vi "sub vi - AI USB4704 (3) v73.vi"(0 "Task0":i32, 1 "Test":bool, 5 "Task1":i32, 7 "Task2":i32, 11 "SAMPLES":dbl, 12 "Max Errors":i32=10, 13 "MAIL SETTINGS":T1) -> (3 "Fault":bool, 4 "data 0":waveform(dbl)[](array[waveform]), 6 "data 1":waveform(dbl)[](array[waveform]), 8 "data 2":waveform(dbl)[](array[waveform]), 10 "loop time":dbl format="%.6g", 14 "Fault Counts":i32[](array[numeric]), 15 "error array":errorcluster[](array[cluster]))   [LabVIEW 2017]
uses:
  <userlib>/DAQNavi Polymorphic VI/read/DAQNavi Read (Analog 1D Wfm NChan NSamp).vi
panel:
  in  "File Path":path
  out "Fault 3":bool
  out "Fault 2":bool
  out "Fault 1":bool
  out "String":string
  in  "Tab Control":enum32{"USB #0", "USB #1", "USB #2"}(tab)
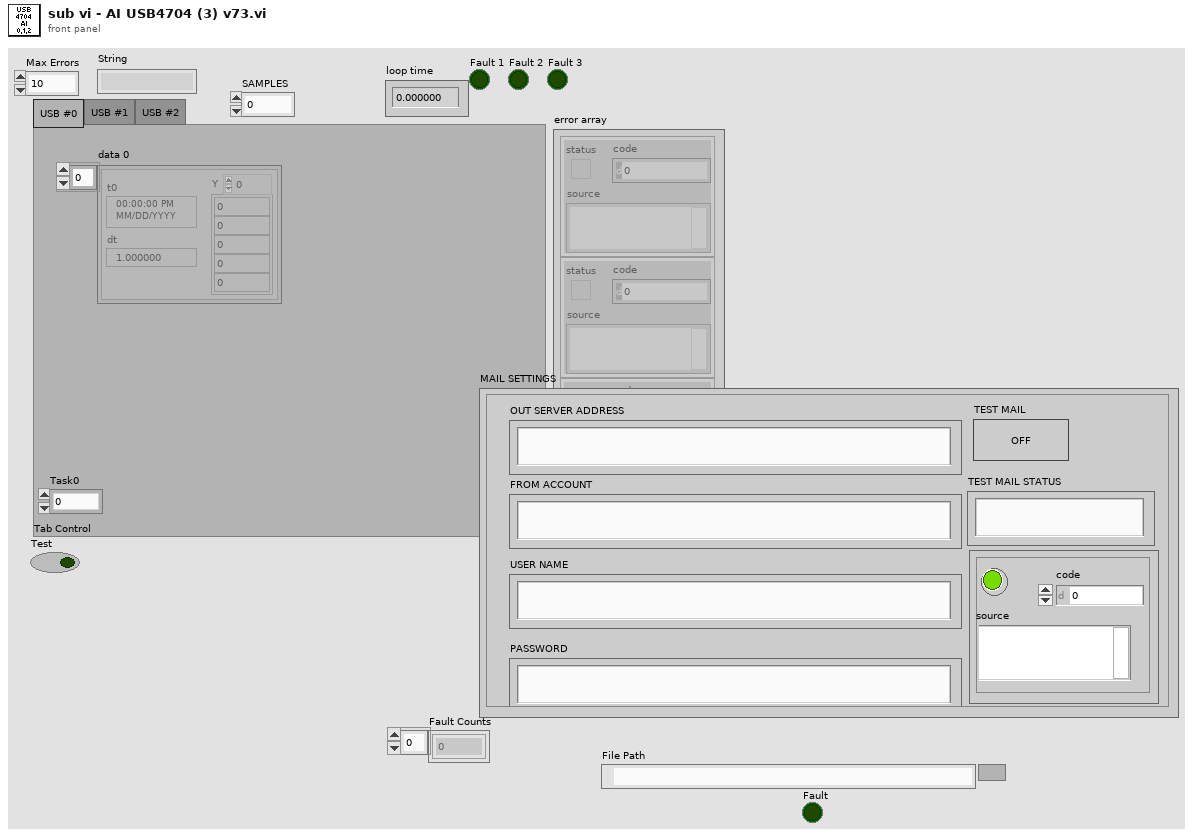
[diagram p1: front panel]
types:
  T1 = cluster{"OUT SERVER ADDRESS":string, "FROM ACCOUNT":string, "USER NAME":string, "PASSWORD":string, "TEST MAIL":bool, "TEST MAIL STATUS":string, "mail error":errorcluster}
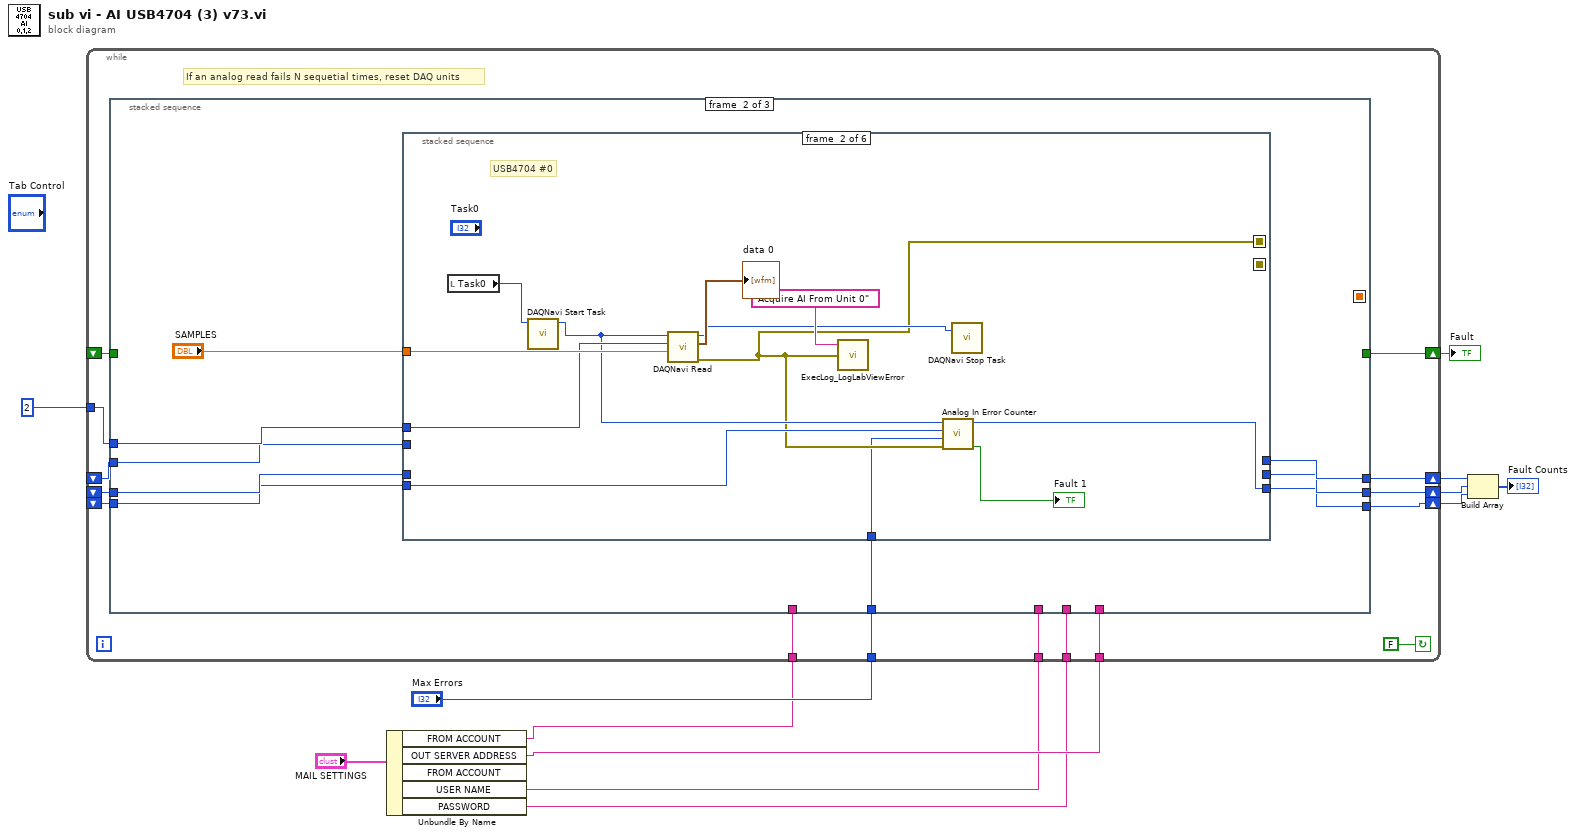
[diagram p0: block diagram]
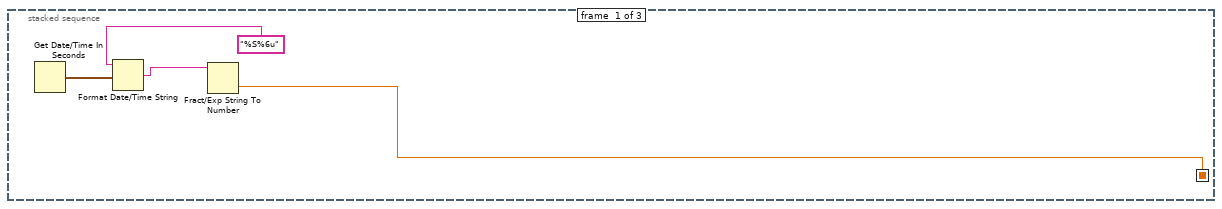
[diagram p2: hidden frame]
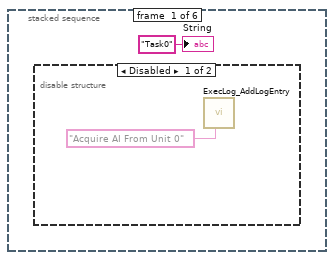
[diagram p3: hidden frame]
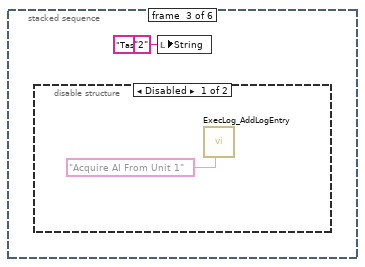
[diagram p5: hidden frame]
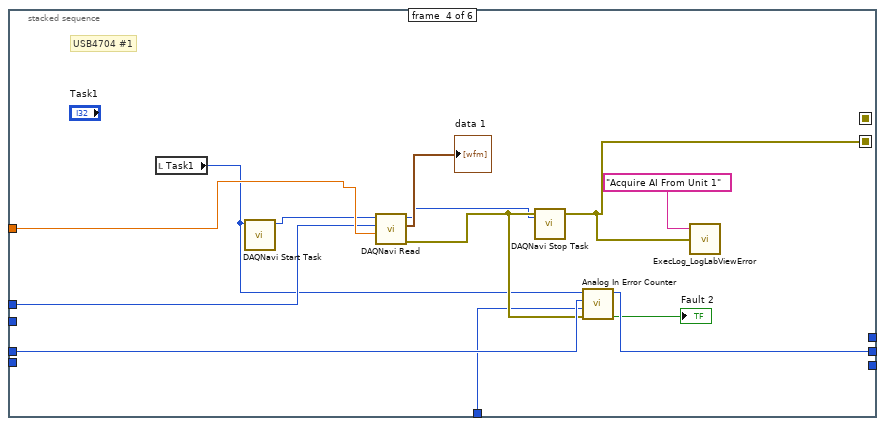
[diagram p7: hidden frame]
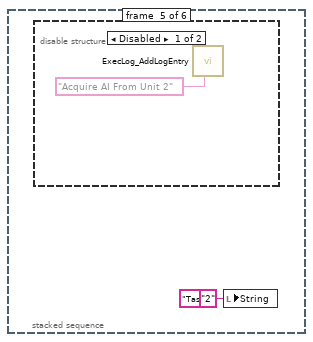
[diagram p8: hidden frame]
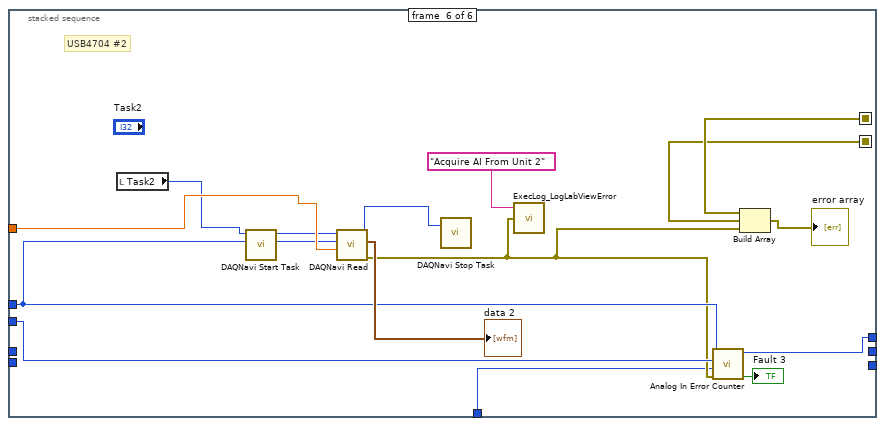
[diagram p10: hidden frame]
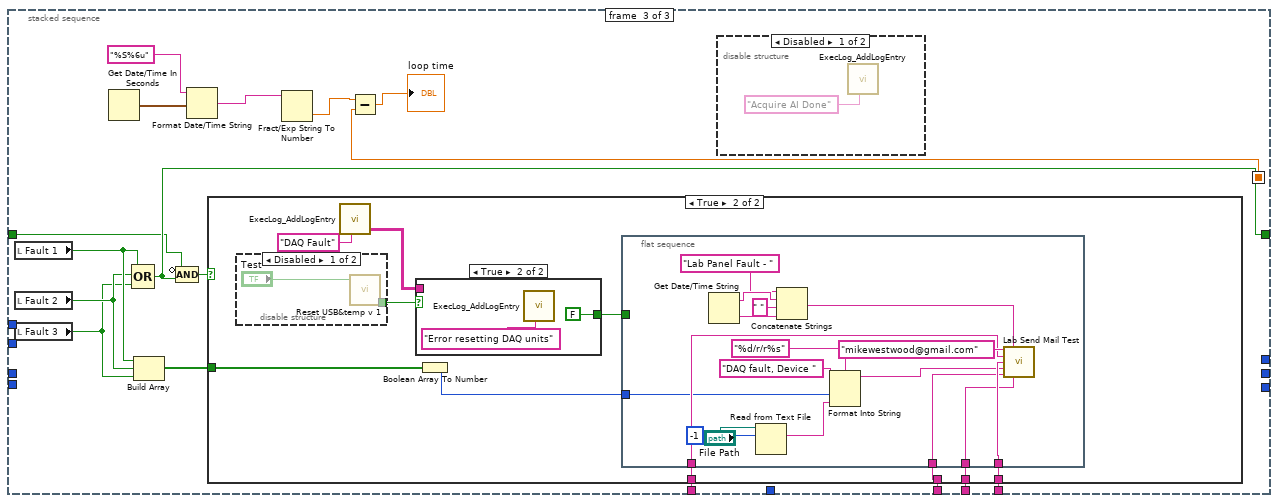
[diagram p11: hidden frame]
diagram:
  n1 = Unbundle By Name("MAIL SETTINGS") -> ("FROM ACCOUNT"=w8:string, "OUT SERVER ADDRESS"=w9:string, "USER NAME"=w7:string, "PASSWORD"=w6:string)  [unwired: 1 out]
  n2 = while {
    tunnel: 2 -> [w27]
    shift-right: [w26] -> w5
    shift-left: _ -> [w25]
    shift-right: [w23] -> w4
    shift-left: _ -> [w24]
    shift-right: [w21] -> w3
    shift-left: _ -> [w22]
    tunnel: "Max Errors" -> [w19]
    tunnel: w9 -> [w18]
    tunnel: w8 -> [w17]
    tunnel: w7 -> [w16]
    tunnel: w6 -> [w15]
    shift-right: [w14] -> w1
    shift-left: _ -> [w13]
    stop <- FALSE continue-if-true
    # "If an analog read fails N sequetial times, reset DAQ units"
    n3 = stacked-sequence {
      seq-local: [w28 _ _] -> [_ _ w100]
      tunnel: w27 -> [_ w40 _]
      tunnel: [_ w38 _] -> w26
      tunnel: w25 -> [_ w37 _]
      tunnel: w24 -> [_ w36 _]
      tunnel: [_ w35 _] -> w23
      tunnel: w22 -> [_ w34 _]
      tunnel: [_ w33 _] -> w21
      tunnel: w19 -> [_ w32 _]
      tunnel: w18 -> [_ _ w98]
      tunnel: w17 -> [_ _ w97]
      tunnel: w16 -> [_ _ w96]
      tunnel: w15 -> [_ _ w95]
      tunnel: [_ _ w90] -> w14
      tunnel: w13 -> [_ _ w88]
      frame #0 {
        n4 = Get Date/Time In Seconds() -> (seconds since 1Jan1904=w30:timestamp)
        n5 = Format Date/Time String(time format string (%c)="%S%6u", seconds (now)=w30) -> (date/time string=w29:string)  [unwired: 1 in]
        n6 = Fract/Exp String To Number(string=w29) -> (number=w28:dbl)  [unwired: 3 in, 1 out]
      }
      frame #1 {
        n7 = stacked-sequence {
          seq-local: [_ w45 _ _ _ _] -> [_ _ _ _ _ w86]
          seq-local: [_ _ _ w62 _ _] -> [_ _ _ _ _ w85]
          tunnel: "SAMPLES" -> [_ w54 _ w69 _ w87]
          tunnel: w40 -> [_ w53 _ w68 _ w80]
          tunnel: [_ _ _ _ _ w81] -> w38
          tunnel: w37 -> [_ _ _ _ _ w82]
          tunnel: w36 -> [_ _ _ w66 _ _]
          tunnel: [_ _ _ w65 _ _] -> w35
          tunnel: w34 -> [_ w51 _ _ _ _]
          tunnel: [_ w50 _ _ _ _] -> w33
          tunnel: w32 -> [_ w44 _ w58 _ w73]
          frame #0 {
            n8 = disable-structure shown="Disabled" {
              frame Disabled {
                n9 = call "ExecLog_AddLogEntry.vi"("Msg"="Acquire AI From Unit 0") -> ()  [unwired: 7 in, 3 out]
              }
              frame Enabled {
              }
            }
            "String" <- "Task0" ("String")
          }
          frame #1 {
            # "USB4704 #0"
            n10 = local read "Task0"() -> (w48:i32)
            n11 = call <userlib>:"DAQNavi Start Task.vi"("task in"=w48) -> ("task out"=w47:i32)  [unwired: 9 in, 1 out]
            n12 = call-poly <userlib>:"DAQNavi Read.vi"("number of samples per channel to read"=w54, "timeout"=w53, "task in"=w47) -> ("error out"=w45:errorcluster, "data"=→"data 0":waveform(dbl)[], "task out"=w46:i32)  [unwired: 1 in, 5 out]
            n13 = call "ExecLog_LogLabViewError.vi"("error IO"=w45, "string 1"="Acquire AI From Unit 0" ("Msg")) -> ()  [unwired: 2 in, 1 out]
            n14 = call "Analog In Error Counter.vi"("error in (no error)"=w45, "Max Errors"=w44, "Count"=w51, "Unit"=w47) -> ("Fault"=→"Fault 1":bool, "Numeric out"=w50:i32)  [unwired: 6 in]
            n15 = call <userlib>:"DAQNavi Stop Task.vi"("task in"=w46) -> ()  [unwired: 1 in, 2 out]
          }
          frame #2 {
            n16 = disable-structure shown="Disabled" {
              frame Disabled {
                n17 = call "ExecLog_AddLogEntry.vi"("Msg"="Acquire AI From Unit 1") -> ()  [unwired: 7 in, 3 out]
              }
              frame Enabled {
              }
            }
            n18 = local write "String"("Task1" ("String")) -> ()
            n19 = local write "String"("2" ("String")) -> ()
          }
          frame #3 {
            # "USB4704 #1"
            n20 = local read "Task1"() -> (w60:i32)
            n21 = call <userlib>:"DAQNavi Start Task.vi"("task in"=w60) -> ("task out"=w59:i32)  [unwired: 9 in, 1 out]
            n22 = call-poly <userlib>:"DAQNavi Read.vi"("number of samples per channel to read"=w69, "timeout"=w68, "task in"=w59) -> ("error out"=w62:errorcluster, "data"=→"data 1":waveform(dbl)[], "task out"=w61:i32)  [unwired: 1 in, 5 out]
            n23 = call <userlib>:"DAQNavi Stop Task.vi"("task in"=w61) -> ()  [unwired: 1 in, 2 out]
            n24 = call "Analog In Error Counter.vi"("error in (no error)"=w62, "Max Errors"=w58, "Count"=w66, "Unit"=w60) -> ("Fault"=→"Fault 2":bool, "Numeric out"=w65:i32)  [unwired: 6 in]
            n25 = call "ExecLog_LogLabViewError.vi"("error IO"=w62, "string 1"="Acquire AI From Unit 1" ("Msg")) -> ()  [unwired: 2 in, 1 out]
          }
          frame #4 {
            n26 = disable-structure shown="Disabled" {
              frame Disabled {
                n27 = call "ExecLog_AddLogEntry.vi"("Msg"="Acquire AI From Unit 2") -> ()  [unwired: 7 in, 3 out]
              }
              frame Enabled {
              }
            }
            n28 = local write "String"("Task2" ("String")) -> ()
            n29 = local write "String"("2" ("String")) -> ()
          }
          frame #5 {
            # "USB4704 #2"
            n30 = local read "Task2"() -> (w76:i32)
            n31 = call <userlib>:"DAQNavi Start Task.vi"("task in"=w76) -> ("task out"=w75:i32)  [unwired: 9 in, 1 out]
            n32 = call-poly <userlib>:"DAQNavi Read.vi"("number of samples per channel to read"=w87, "timeout"=w80, "task in"=w75) -> ("error out"=w77:errorcluster, "data"=→"data 2":waveform(dbl)[], "task out"=w74:i32)  [unwired: 1 in, 5 out]
            n33 = call <userlib>:"DAQNavi Stop Task.vi"("task in"=w74) -> ()  [unwired: 1 in, 2 out]
            n34 = call "ExecLog_LogLabViewError.vi"("error IO"=w77, "string 1"="Acquire AI From Unit 2" ("Msg")) -> ()  [unwired: 2 in, 1 out]
            n35 = call "Analog In Error Counter.vi"("error in (no error)"=w77, "Max Errors"=w73, "Count"=w82, "Unit"=w80) -> ("Fault"=→"Fault 3":bool, "Numeric out"=w81:i32)  [unwired: 6 in]
            n36 = Build Array(w86, w85, w77) -> (→"error array":errorcluster[])
          }
        }
      }
      frame #2 {
        n37 = local read "Fault 1"() -> (w94:bool)
        n38 = local read "Fault 2"() -> (w93:bool)
        n39 = local read "Fault 3"() -> (w92:bool)
        n40 = Get Date/Time In Seconds() -> (seconds since 1Jan1904=w103:timestamp)
        n41 = Compound Arithmetic op=OR(w94, w93, w92) -> (w90:bool)
        n42 = Build Array(w94, w93, w92) -> (w91:bool[])
        n43 = Compound Arithmetic op=AND(invert w88, w90) -> (w89:bool)
        n44 = Format Date/Time String(time format string (%c)="%S%6u", seconds (now)=w103) -> (date/time string=w102:string)  [unwired: 1 in]
        n45 = case shown="True" w89 {
          tunnel: w98 -> [_ w114]
          tunnel: w97 -> [_ w113]
          tunnel: w96 -> [_ w112]
          tunnel: w95 -> [_ w111]
          tunnel: w91 -> [_ w110]
          frame False {
          }
          frame True {
            n46 = disable-structure shown="Disabled" {
              disable-tunnel: [w116 _] -> w115
              frame Disabled {
                n47 = call "Reset USB&temp v 1.vi"("Test"="Test") -> ("Reset Error"=w116:bool)  [unwired: 10 in]
              }
              frame Enabled {
              }
            }
            n48 = call "ExecLog_AddLogEntry.vi"("Msg"="DAQ Fault") -> ("Log"=w107:string[][])  [unwired: 7 in, 2 out]
            n49 = case shown="True" w115 {
              tunnel: w107 -> [_ _]
              tunnel: [_ FALSE] -> w106
              frame False {
              }
              frame True {
                n50 = call "ExecLog_AddLogEntry.vi"("Msg"="Error resetting DAQ units" ("message")) -> ()  [unwired: 7 in, 3 out]
              }
            }
            n51 = Boolean Array To Number(Boolean array=w110) -> (number=w109:u32)
            n52 = flat-sequence {
              tunnel: w114 -> [w133]
              tunnel: w113 -> [w132]
              tunnel: w112 -> [w129]
              tunnel: w111 -> [w128]
              tunnel: w109 -> [w123]
              tunnel: w106 -> [_]
              frame #0 {
                n53 = Get Date/Time String() -> (date string=w131:string, time string=w130:string)  [unwired: 3 in]
                n54 = Read from Text File(file (use dialog)="File Path", count=-1) -> (text=w120:string)  [unwired: 2 in, 3 out]
                n55 = Concatenate Strings("Lab Panel Fault - " ("string"), w131, " " ("string"), w130) -> (w125:string)
                n56 = Format Into String(format string="%d/r/r%s", initial string="DAQ fault, Device " ("message"), w123, w120) -> (resulting string=w122:string)  [unwired: 1 in, 1 out]
                n57 = call "Lab Send Mail Test.vi"("TO:"="mikewestwood@gmail.com", "subject"=w125, "from"=w132, "out going server"=w133, "message"=w122, "username"=w129, "password"=w128) -> ()  [unwired: 8 in, 1 out]
              }
            }
          }
        }
        n58 = Fract/Exp String To Number(string=w102) -> (number=w101:dbl)  [unwired: 3 in, 1 out]
        n59 = Subtract(x=w101, y=w100) -> (x-y=→"loop time":dbl)
        n60 = disable-structure shown="Disabled" {
          frame Disabled {
            n61 = call "ExecLog_AddLogEntry.vi"("Msg"="Acquire AI Done") -> ()  [unwired: 7 in, 3 out]
          }
          frame Enabled {
          }
        }
      }
    }
  }
  "Fault" <- w1
  n62 = Build Array(w5, w4, w3) -> (→"Fault Counts":i32[])
